vi "displaydaqwave.vi"(8 "Samples per Waveform":u32=95, 9 "Location":i16(ring) items=["Purdue", "NIKHEF", "Zurich", "???"], 10 "Trigger level":i16[](array[numeric])=[4000, 4000, 4000, 4000, 4000, 4000, 4000, 4000] caption="Trigger", 11 "Waveform from DAQ":i16[](array[numeric])) -> (0 "Waveform Graph":dynamicdata(graph), 3 "Channel number displayed":i16=-1)   [LabVIEW 2012]
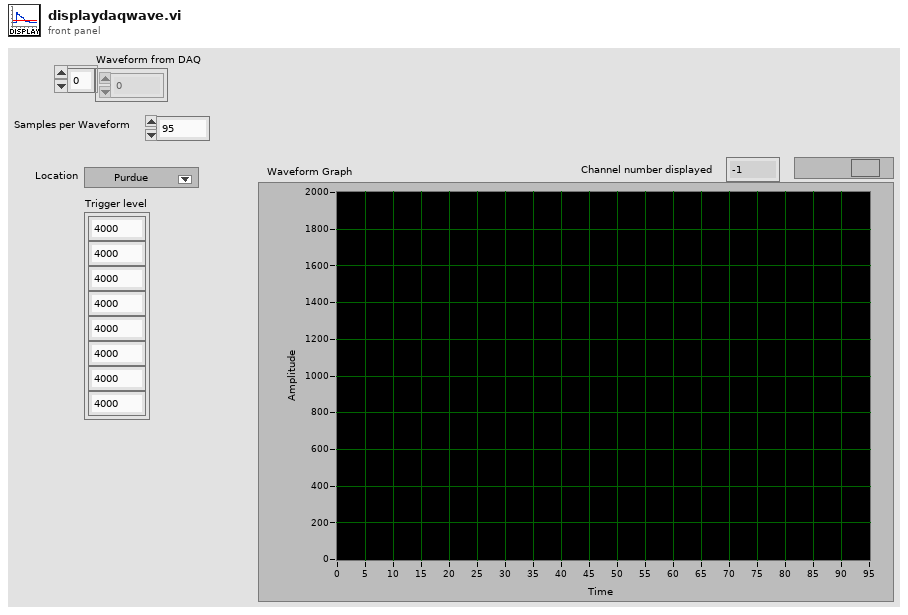
[diagram p1: front panel]
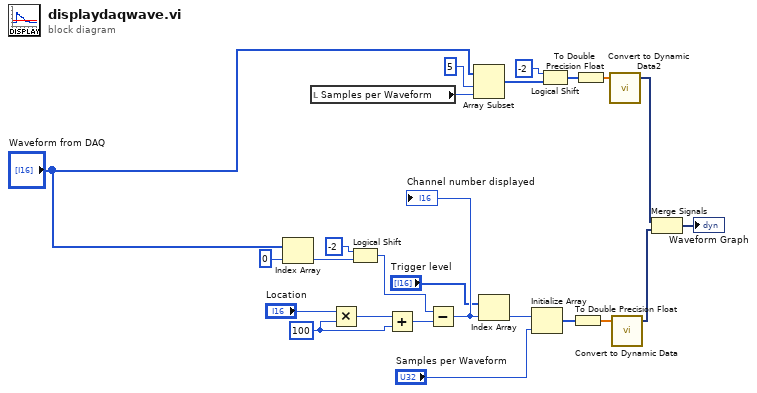
[diagram p0: block diagram]
diagram:
  w11 = i16 100
  n1 = Index Array(array="Waveform from DAQ", index=0) -> (element=w1:i16)
  n2 = local read "Samples per Waveform"() -> (w23:u32)
  n3 = Multiply(x="Location", y=w11) -> (x*y=w12:i16)
  n4 = Logical Shift(y=i16 -2, x=w1) -> (x << y=w15:i16)
  n5 = Add(x=w12, y=w11) -> (x+y=w13:i16)
  n6 = Subtract(x=w15, y=w13) -> (x-y=w5:i16)
  "Channel number displayed" <- w5
  n7 = Array Subset(array="Waveform from DAQ", index=5, length=w23) -> (w20:i16[])
  n8 = Index Array(array="Trigger level", index=w5) -> (element=w9:i16)
  n9 = Initialize Array(w9, "Samples per Waveform") -> (w6:i16[])
  n10 = Logical Shift(y=i16 -2, x=w20) -> (x << y=w19:i16[])
  n11 = To Double Precision Float(number=w6) -> (double precision float=w10:dbl[])
  n12 = To Double Precision Float(number=w19) -> (double precision float=w22:dbl[])
  n13 = call "Convert to Dynamic Data2"("Array"=w22) -> ("Dynamic Data Type"=w17:dynamicdata)  [unwired: 3 in]
  n14 = call "Convert to Dynamic Data"("Array"=w10) -> ("Dynamic Data Type"=w7:dynamicdata)  [unwired: 3 in]
  n15 = Merge Signals(w17, w7) -> (→"Waveform Graph":dynamicdata)
